vi "Write Read Instrument.vi"(7 "Language Selector (-1)":i16(ring)=-1 items=["none"=-1, "GEN"=0, "SCPI"=1], 8 "error in (no error)":errorcluster, 9 "GEN  Write Command/Query":string, 10 "SCPI  Write Command/Query":string, 11 "VISA resource name":refnum<visa-resource-name>) -> (0 "error out":errorcluster, 2 "Response":string, 3 "VISA resource name out":refnum<visa-resource-name>)   [LabVIEW 2018, in "TDK-Lambda Z.lvlib"]
doc: "This VI sends any SCPI or GEN command to the Z+ power supply \nIf command returns error (from the instrument's SYST:ERR queue), the VI path, command string and SYST:ERR message are added to the \"error out\" string.\nThis VI sends any SCPI or GEN query to the Z+ and reads the response message. The Return Count is the number of characters read.\nIf a query error occurs, such as no response message because the query is illegal, the system error (SYST:ERR?) is read and returned in the \"error out\" cluster\n\n\nNote:\nIncludes error checking after query sent. Adds checksum to query string"
uses:
  TDK-Lambda Z.lvlib
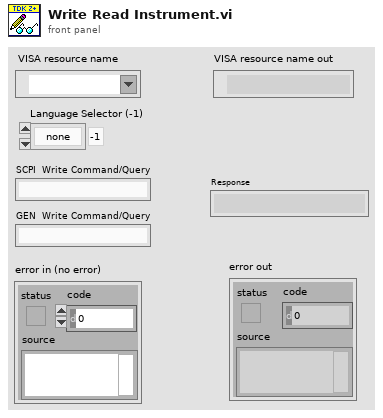
[diagram p1: front panel]
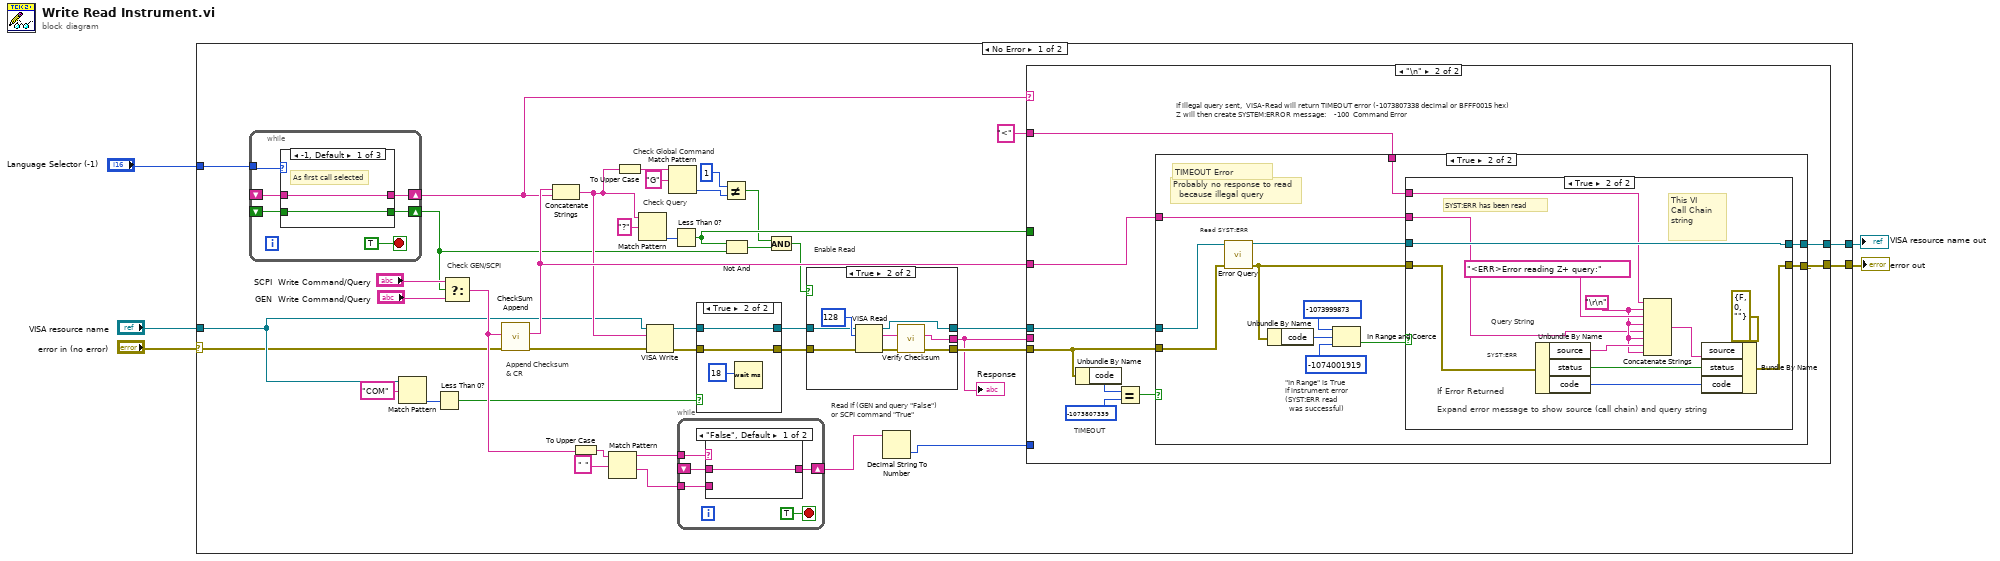
[diagram p0: block diagram]
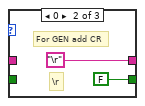
[diagram p3: hidden frame]
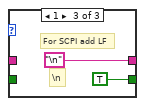
[diagram p4: hidden frame]
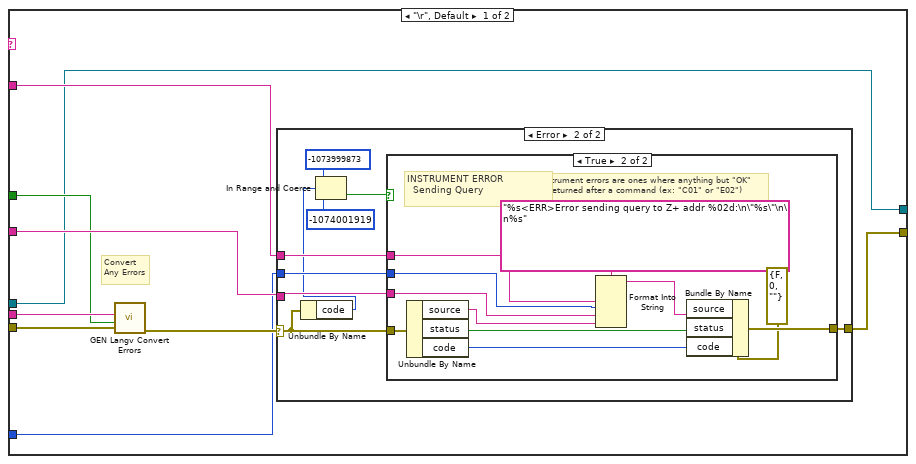
[diagram p6: hidden frame]
diagram:
  n1 = case shown="No Error" "error in (no error)" {
    selector: "error in (no error)" -> [w6 w148]
    tunnel: "VISA resource name" -> [w9 w149]
    tunnel: [w43 w149] -> w4
    tunnel: [w42 w148] -> w3
    tunnel: "Language Selector (-1)" -> [w8 _]
    frame No Error {
      # "Check Global Command"
      # "Append Checksum \n& CR"
      # "Enable Read"
      # "Check GEN/SCPI"
      # "Check Query"
      # "Read If (GEN and query \"False\")\nor SCPI command \"True\""
      n2 = while {
        shift-right: [w58] -> w11
        shift-left: _ -> [w57]
        shift-right: [w55] -> w12
        shift-left: _ -> [w54]
        tunnel: w8 -> [w53]
        stop <- TRUE stop-if-true
        n3 = case shown="-1, Default" w53 {
          tunnel: [w60 "\r" "\n"] -> w58
          tunnel: w57 -> [w60 _ _]
          tunnel: [w59 FALSE TRUE] -> w55
          tunnel: w54 -> [w59 _ _]
          frame -1, Default {
            # "As first call selected"
          }
          frame 0 {
            # "\\r"
            # "For GEN add CR"
          }
          frame 1 {
            # "\\n"
            # "For SCPI add LF"
          }
        }
      }
      n4 = Match Pattern(string=w9, regular expression="COM") -> (offset past match=w16:i32)  [unwired: 1 in, 3 out]
      n5 = Less Than 0?(x=w16) -> (x < 0?=w15:bool)
      n6 = Select(t="SCPI  Write Command/Query", s=w12, f="GEN  Write Command/Query") -> (s? t:f=w29:string)
      n7 = call "CheckSum Append.vi"("error in (no error)"=w6, "Input Cmd"=w29) -> ("error out"=w7:errorcluster, "ChkSum Cmd"=w28:string)  [unwired: 8 in]
      n8 = Concatenate Strings(w28, w11) -> (w13:string)
      n9 = To Upper Case(1:w29) -> (0:w38:string)
      n10 = Match Pattern(string=w38, regular expression=" ") -> (before substring=w36:string, after substring=w10:string)  [unwired: 1 in, 2 out]
      n11 = To Upper Case(1:w13) -> (0:w26:string)
      n12 = Match Pattern(string=w13, regular expression="?") -> (offset past match=w44:i32)  [unwired: 1 in, 3 out]
      n13 = VISA Write(VISA resource name=w9, write buffer=w13, error in (no error)=w7) -> (VISA resource name out=w19:refnum<visa-resource-name>, error out=w21:errorcluster)  [unwired: 1 out]
      n14 = Match Pattern(string=w26, regular expression="G") -> (offset past match=w25:i32)  [unwired: 1 in, 3 out]
      n15 = Less Than 0?(x=w44) -> (x < 0?=w33:bool)
      n16 = while {
        tunnel: w36 -> [w50]
        shift-right: [w48] -> w35
        shift-left: _ -> [w49]
        tunnel: w10 -> [w46]
        stop <- TRUE stop-if-true
        n17 = case shown="\"False\", Default" w50 {
          tunnel: w49 -> [w51 _]
          tunnel: [w51 w52] -> w48
          tunnel: w46 -> [_ w52]
          frame "False", Default {
          }
          frame "ADR", "INST:NSEL" {
          }
        }
      }
      n18 = case shown="True" w15 {
        tunnel: w21 -> [w65 w69]
        tunnel: [w65 w69] -> w20
        tunnel: w19 -> [w66 w68]
        tunnel: [w66 w68] -> w18
        frame False {
        }
        frame True {
          n19 = Wait (ms)(milliseconds to wait=u32 18) -> ()  [unwired: 1 out]
        }
      }
      n20 = Not Equal?(x=1, y=w25) -> (x != y?=w24:bool)
      n21 = Not And(1:w12, 2:w33) -> (0:w23:bool)
      n22 = And(x=w24, y=w23) -> (x .and. y?=w22:bool)
      n23 = case shown="True" w22 {
        tunnel: w20 -> [w138 w146]
        tunnel: w18 -> [w139 w145]
        tunnel: [w139 w140] -> w32
        tunnel: [w138 w141] -> w31
        tunnel: [_ w142] -> w30
        frame False {
        }
        frame True {
          n24 = VISA Read(VISA resource name=w145, byte count=u32 128 ("byte count (0)"), error in (no error)=w146) -> (VISA resource name out=w140:refnum<visa-resource-name>, read buffer=w143:string, error out=w144:errorcluster)  [unwired: 1 out]
          n25 = call "Verify Checksum.vi"("error in (no error)"=w144, "Input Cmd"=w143) -> ("error out"=w141:errorcluster, "Trimmed String"=w142:string)  [unwired: 6 in]
        }
      }
      "Response" <- w30
      n26 = Decimal String To Number(string=w35) -> (number=w34:i32)  [unwired: 2 in, 1 out]
      n27 = case shown="\"\\n\"" w11 {
        tunnel: w31 -> [w77 w106]
        tunnel: w32 -> [w70 w105]
        tunnel: w28 -> [w75 w104]
        tunnel: [w70 w103] -> w43
        tunnel: [w74 w102] -> w42
        tunnel: w30 -> [w78 _]
        tunnel: "<" -> [w73 w101]
        tunnel: w34 -> [w72 _]
        tunnel: w33 -> [w71 _]
        frame "\r", Default {
          # "Convert\nAny Errors"
          n28 = call "GEN Langv Convert Errors.vi"("error in (no error)"=w77, "Expect \"OK\" (F)"=w71, "String in"=w78) -> ("error out"=w76:errorcluster)  [unwired: 8 in]
          n29 = case shown="Error" w76 {
            selector: w76 -> [w79 w82]
            tunnel: w75 -> [_ w87]
            tunnel: [w79 w88] -> w74
            tunnel: w73 -> [_ w86]
            tunnel: w72 -> [_ w85]
            frame No Error {
              # "Query Sent Correctly \n  and response Returned"
            }
            frame Error {
              n30 = Unbundle By Name(w82) -> ("code"=w81:i32)
              n31 = In Range and Coerce(upper limit=-1073999873 ("code"), x=w81, lower limit=-1074001919 ("code")) -> (In Range?=w80:bool)  [unwired: 1 out]
              n32 = case shown="True" w80 {
                tunnel: w82 -> [w89 w100]
                tunnel: [w89 w97] -> w88
                tunnel: w87 -> [_ w95]
                tunnel: w86 -> [_ w92]
                tunnel: w85 -> [_ w91]
                frame False {
                  # "VISA  ERROR  \n  Sending Command"
                  # "For VISA error, do not change error message"
                }
                frame True {
                  # "Instrument errors are ones where anything but \"OK\"\nis returned after a command (ex: \"C01\" or \"E02\")"
                  # "INSTRUMENT ERROR  \n  Sending Query"
                  n33 = Unbundle By Name(w100) -> ("source"=w94:string, "status"=w98:bool, "code"=w99:i32)
                  n34 = Format Into String(format string="%s<ERR>Error sending query to Z+ addr %02d:\n\"%s\"\n\n%s" ("Source"), w92, w91, w95, w94) -> (resulting string=w93:string)  [unwired: 2 in, 1 out]
                  n35 = Bundle By Name(cluster=errorcluster {"status"=FALSE, "code"=0, "source"=""} ("error out 2"), "source"=w93, "status"=w98, "code"=w99) -> (w97:errorcluster)
                }
              }
            }
          }
        }
        frame "\n" {
          # "TIMEOUT"
          # "If illegal query sent,  VISA-Read will return TIMEOUT error (-1073807338 decimal or BFFF0015 hex) \nZ will then create SYSTEM:ERROR message:    -100  Command Error"
          n36 = Unbundle By Name(w106) -> ("code"=w107:i32)
          n37 = Equal?(x=w107, y=-1073807339 ("code")) -> (x = y?=w109:bool)
          n38 = case shown="True" w109 {
            tunnel: [w110 w122] -> w102
            tunnel: [w111 w123] -> w103
            tunnel: w105 -> [w111 w114]
            tunnel: w106 -> [w110 w112]
            tunnel: w104 -> [_ w115]
            tunnel: w101 -> [_ w113]
            frame False {
              # "Maybe some other VISA error,  pass it out\nIf error occurred, , \"Response\" is empty and \"Return Count\" is zero"
              # "Not TIMEOUT Error (maybe successful query)"
            }
            frame True {
              # "\"In Range\" is True\nif instrument error\n(SYST:ERR read\n  was successful)"
              # "TIMEOUT Error"
              # "Probably no response to read  \n  because illegal query"
              # "Read SYST:ERR"
              n39 = call "Error Query.vi"("error in (no error)"=w112, "VISA resource name"=w114) -> ("error out"=w117:errorcluster, "VISA resource name out"=w116:refnum<visa-resource-name>)  [unwired: 6 in, 2 out]
              n40 = Unbundle By Name(w117) -> ("code"=w118:i32)
              n41 = In Range and Coerce(upper limit=-1073999873 ("code"), x=w118, lower limit=-1074001919 ("code")) -> (In Range?=w119:bool)  [unwired: 1 out]
              n42 = case shown="True" w119 {
                tunnel: w117 -> [w125 w131]
                tunnel: [w125 w132] -> w122
                tunnel: w116 -> [w124 w130]
                tunnel: [w124 w130] -> w123
                tunnel: w115 -> [_ w128]
                tunnel: w113 -> [_ w126]
                frame False {
                  # "Read SYST:ERR returned VISA communication error.\n  Comm is dead,  just pass error out"
                }
                frame True {
                  w129 = "\r\n"
                  # "This VI \nCall Chain \nstring"
                  # "Query String"
                  # "Expand error message to show source (call chain) and query string"
                  # "SYST:ERR"
                  # "If Error Returned"
                  # "SYST:ERR has been read"
                  n43 = Unbundle By Name(w131) -> ("source"=w134:string, "status"=w136:bool, "code"=w135:i32)
                  n44 = Concatenate Strings(w126, w129, "<ERR>Error reading Z+ query:" ("Source"), w129, w128, w129, w134, w129) -> (w137:string)
                  n45 = Bundle By Name(cluster=errorcluster {"status"=FALSE, "code"=0, "source"=""} ("error out 2"), "source"=w137, "status"=w136, "code"=w135) -> (w132:errorcluster)
                }
              }
            }
          }
        }
      }
    }
    frame Error {
    }
  }
  "VISA resource name out" <- w4
  "error out" <- w3
